vi "extractTaskRefTerminal.vi"(8 "error in (no error)":errorcluster, 11 "VI in":refnum<vi>) -> (0 "error out":errorcluster, 1 "found?":bool, 2 "taskRefTerminal":refnum<vi>, 3 "VI out":refnum<vi>)   [LabVIEW 2023]
uses:
  <vilib>/Utility/traverseref.llb/TRef TravTarget.ctl
  <vilib>/Utility/traverseref.llb/VI Scripting - Traverse.lvlib
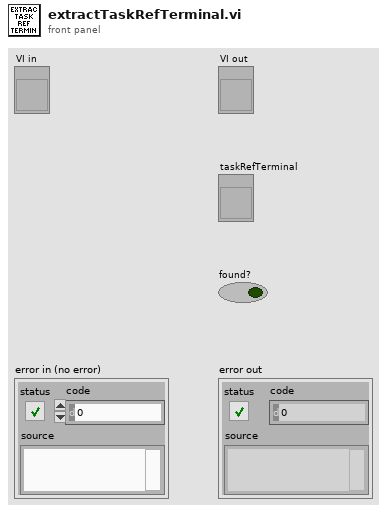
[diagram p1: front panel]
types:
  T1 = typedef "TRef TravTarget.ctl" = enum16{"FP", "BD", "Other"}
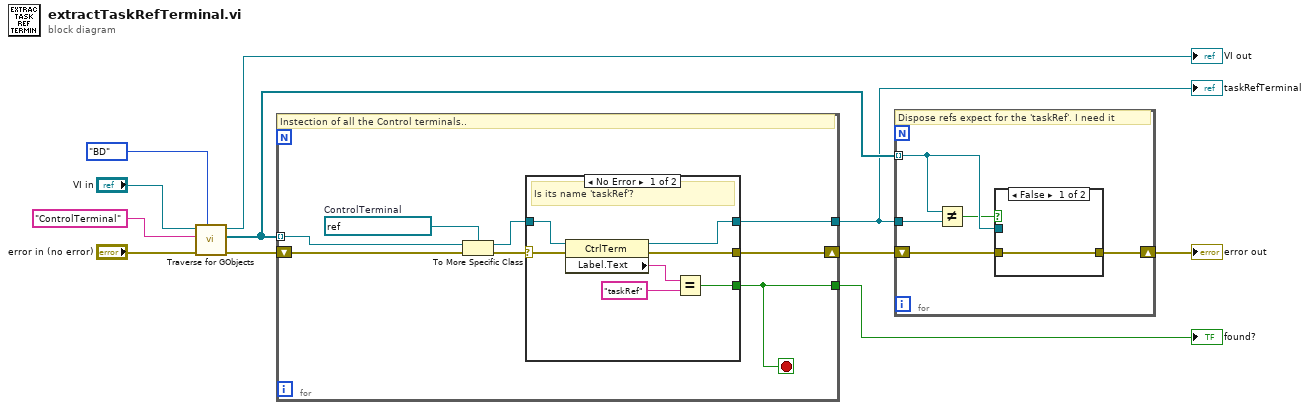
[diagram p0: block diagram]
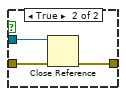
[diagram p2: hidden frame]
diagram:
  n1 = call <vilib>:"Traverse for GObjects.vi"("Traverse Target"=TRef_TravTarget."BD", "error in (no error)"="error in (no error)", "Class Name"="ControlTerminal", "VI Refnum"="VI in") -> ("error out"=w10:errorcluster, "References"=w4:refnum<vi>[], "dup VI Refnum"=→"VI out":refnum<vi>)  [unwired: 4 in, 1 out]
  n2 = for {
    tunnel: w4 -> [w12] mode=indexing
    shift-right: [w15] -> w3
    shift-left: w10 -> [w16]
    tunnel: [w14] -> w1
    tunnel: [w13] -> w11
    stop <- w13 stop-if-true
    w17 = refnum<vi> refnum  # ControlTerminal
    # "Instection of all the Control terminals.."
    n3 = To More Specific Class(target class=w17, reference=w12, error in=w16) -> (specific class reference=w18:refnum<vi>, error out=w19:errorcluster)
    n4 = case shown="No Error" w19 {
      selector: w19 -> [w26 _]
      tunnel: w18 -> [w25 _]
      tunnel: [w24 _] -> w15
      tunnel: [w21 _] -> w13
      tunnel: [w20 _] -> w14
      frame No Error {
        # "Is its name 'taskRef'?"
        n5 = property class="CtrlTerm"(reference=w25, error in=w26) -> (reference out=w20:refnum<vi>, error out=w24:errorcluster, "Label.Text"=w23:string)
        n6 = Equal?(x=w23, y="taskRef") -> (x = y?=w21:bool)
      }
      frame Error {
      }
    }
  }
  "taskRefTerminal" <- w1
  "found?" <- w11
  n7 = for {
    shift-right: [w30] -> w2
    shift-left: w3 -> [w31]
    tunnel: w4 -> [w29] mode=indexing
    tunnel: w1 -> [w28]
    # "Dispose refs expect for the 'taskRef'. I need it"
    n8 = Not Equal?(x=w29, y=w28) -> (x != y?=w27:bool)
    n9 = case shown="False" w27 {
      tunnel: w31 -> [w32 w35]
      tunnel: [w32 w34] -> w30
      tunnel: w29 -> [_ w33]
      frame False {
      }
      frame True {
        n10 = Close Reference(reference=w33, error in (no error)=w35) -> (error out=w34:errorcluster)
      }
    }
  }
  "error out" <- w2
